vi "FTW-Image-ToPicture.vi"(1 "Image":T1) -> (0 "Picture":picture)   [LabVIEW 2013]
doc: "Draws a 1-, 4-, or 8-bit pixmap or a 24-bit RGB pixmap into a picture."
panel:
  # "Inputs"
  # "Outputs"
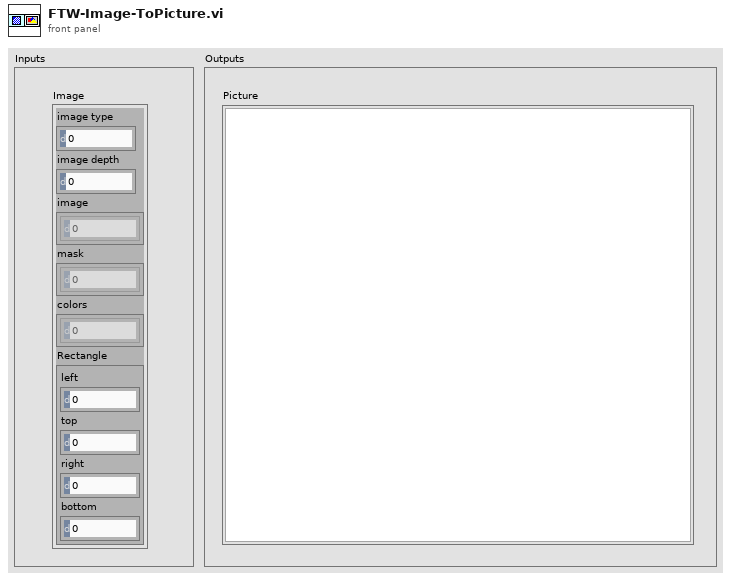
[diagram p1: front panel]
types:
  T1 = cluster{"image type":i32, "image depth":i32, "image":u8[], "mask":u8[], "colors":u32[], "Rectangle":cluster{"left":i16, "top":i16, "right":i16, "bottom":i16}}
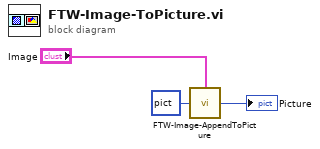
[diagram p0: block diagram]
diagram:
  n1 = call "FTW-Image-AppendToPicture.vi"("Image"="Image", "Initial Picture"=picture data[5B]) -> ("Picture"=→"Picture":picture)  [unwired: 2 in]
